vi "From Control Value to Command.vi"(4 "Maximum Speed":u8=100 max=100, 6 "Servo?":bool, 7 "Command Beginning":u32=16716064 format="%x", 8 "Error In":errorcluster, 11 "From -100 to 100":i8 min=-100 max=100) -> (0 "Error Out":errorcluster, 3 "Command in Hex":u32 format="%x")   [LabVIEW 2014]
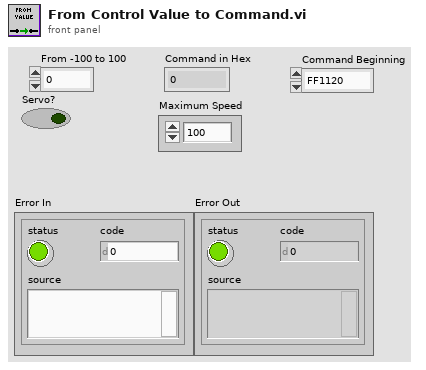
[diagram p1: front panel]
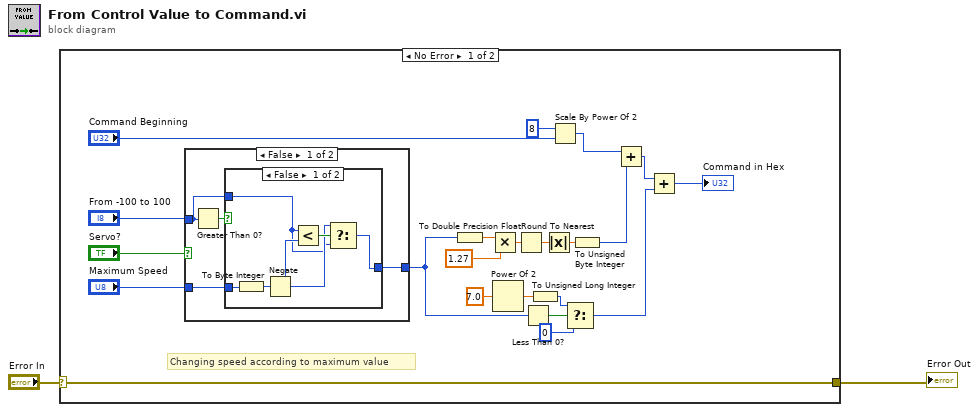
[diagram p0: block diagram]
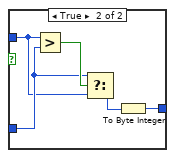
[diagram p2: hidden frame]
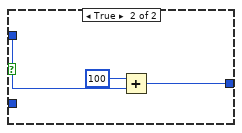
[diagram p3: hidden frame]
diagram:
  n1 = case shown="No Error" "Error In" {
    selector: "Error In" -> [w17 w43]
    tunnel: [w17 w43] -> w1
    frame No Error {
      # "Changing speed according to maximum value"
      n2 = case shown="False" "Servo?" {
        tunnel: [w25 w40] -> w6
        tunnel: "From -100 to 100" -> [w27 w42]
        tunnel: "Maximum Speed" -> [w26 _]
        frame False {
          n3 = Greater Than 0?(x=w27) -> (x > 0?=w28:bool)
          n4 = case shown="False" w28 {
            tunnel: w27 -> [w30 w37]
            tunnel: w26 -> [w33 w38]
            tunnel: [w29 w36] -> w25
            frame False {
              n5 = To Byte Integer(number=w33) -> (8bit integer=w34:i8)
              n6 = Negate(x=w34) -> (-x=w31:i8)
              n7 = Less?(x=w30, y=w31) -> (x < y?=w32:bool)
              n8 = Select(t=w31, s=w32, f=w30) -> (s? t:f=w29:i8)
            }
            frame True {
              n9 = Greater?(x=w37, y=w38) -> (0:w39:bool)
              n10 = Select(t=w38, s=w39, f=w37) -> (s? t:f=w35:u8)
              n11 = To Byte Integer(number=w35) -> (8bit integer=w36:i8)
            }
          }
        }
        frame True {
          n12 = Add(x=i8 100, y=w42) -> (x+y=w40:i16)
        }
      }
      n13 = To Double Precision Float(number=w6) -> (double precision float=w12:dbl)
      n14 = Multiply(x=w12, y=1.27) -> (x*y=w14:dbl)
      n15 = Power Of 2(x=7.0) -> (2^x=w8:dbl)
      n16 = Round To Nearest(number=w14) -> (nearest integer value=w15:dbl)
      n17 = Less Than 0?(x=w6) -> (x < 0?=w9:bool)
      n18 = To Unsigned Long Integer(number=w8) -> (unsigned 32bit integer=w10:u32)
      n19 = Absolute Value(x=w15) -> (abs(x)=w16:dbl)
      n20 = Scale By Power Of 2(n=i16 8, x="Command Beginning") -> (x*2^n=w24:u32)
      n21 = Select(t=w10, s=w9, f=u32 0) -> (s? t:f=w19:u32)
      n22 = To Unsigned Byte Integer(number=w16) -> (unsigned 8bit integer=w18:u8)
      n23 = Add(x=w24, y=w18) -> (x+y=w20:u32)
      n24 = Add(x=w20, y=w19) -> (x+y=→"Command in Hex":u32)
    }
    frame Error {
    }
  }
  "Error Out" <- w1
